vi "BME_DG_Set_G02_Chnl.vi"(8 "error in (no error)":errorcluster, 9 "ChnParemater":T1 {"Delay (µs)" min=0.0 max=100000000.0 format="%.5f"}, 10 "Channel":u32=1, 11 "DG_Number":i32) -> (0 "error out":errorcluster, 3 "return code":i32)   [LabVIEW 2009, in "POLARIS BME DG.lvlib"]
uses:
  POLARIS BME DG.lvlib
  ChnlSettings.ctl
  BME DLL/DelayGenerator.dll
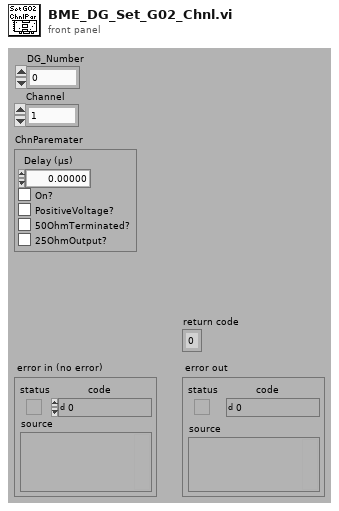
[diagram p1: front panel]
types:
  T1 = typedef "POLARIS BME DG.lvlib/ChnlSettings.ctl" = cluster{" Delay (µs)":dbl, "On?":bool, "PositiveVoltage?":bool, "50OhmTerminated? ":bool, "25OhmOutput?":bool}
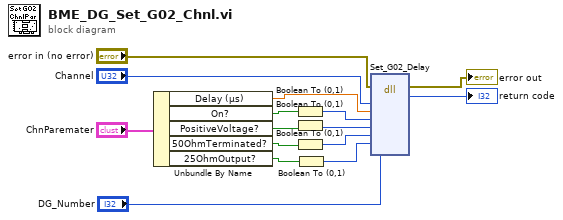
[diagram p0: block diagram]
diagram:
  n1 = Unbundle By Name("ChnParemater") -> ("Delay (µs)"=w8:dbl, "On?"=w7:bool, "PositiveVoltage?"=w6:bool, "50OhmTerminated?"=w5:bool, "25OhmOutput?"=w4:bool)
  n2 = Boolean To (0,1)(Boolean=w7) -> (0, 1=w14:i16)
  n3 = Boolean To (0,1)(Boolean=w6) -> (0, 1=w13:i16)
  n4 = Boolean To (0,1)(Boolean=w5) -> (0, 1=w12:i16)
  n5 = Boolean To (0,1)(Boolean=w4) -> (0, 1=w11:i16)
  n6 = dll-call lib="G:/CSPOLARIS Updates/POLARIS BME DG/BME DLL/DelayGenerator.dll" fn="Set_G02_Delay"(error in="error in (no error)", "Channel"="Channel", "FireFirst"=w8, "Active"=w14, "Positive"=w13, "Terminate"=w12, "HighDrive"=w11, "DG_Number"="DG_Number") -> (error out=→"error out":errorcluster, "return code"=→"return code":i32)  [unwired: 9 in, 1 out]
